vi "DataSetToVariantArrays.vi"() -> ()   [LabVIEW 2014, in "TableLogger_SQLite_Actor.lvlib" / "TableLogger_SQLite_Actor.lvclass"]
uses:
  TableLogger_SQLite_Actor.lvclass
  TableLogger_Actor/TableLogger_Actor/TableLogger_Actor.lvclass
panel:
  out "Data 2":variant[](array[variant])
  out "Data":string[](array[string])
  in  "LV Data":T1={"Numeric Data"=1245, "Float Data"=896.578, "String Data"="Tessolve", "Enum Data"=enum."Enum Item 2", "Array Data"=[8787, 457], "Cluster"={"String"="Hi", "Array Data 2"=[1, 2]}, "Array Data 2"=[3, 2, 1], "Cluster 2"={"String"="hello", "Array Data 2"=[1, 2]}, "Cluster 3"={"Cluster78"={"Array Data 2"=[987, 789]}}}
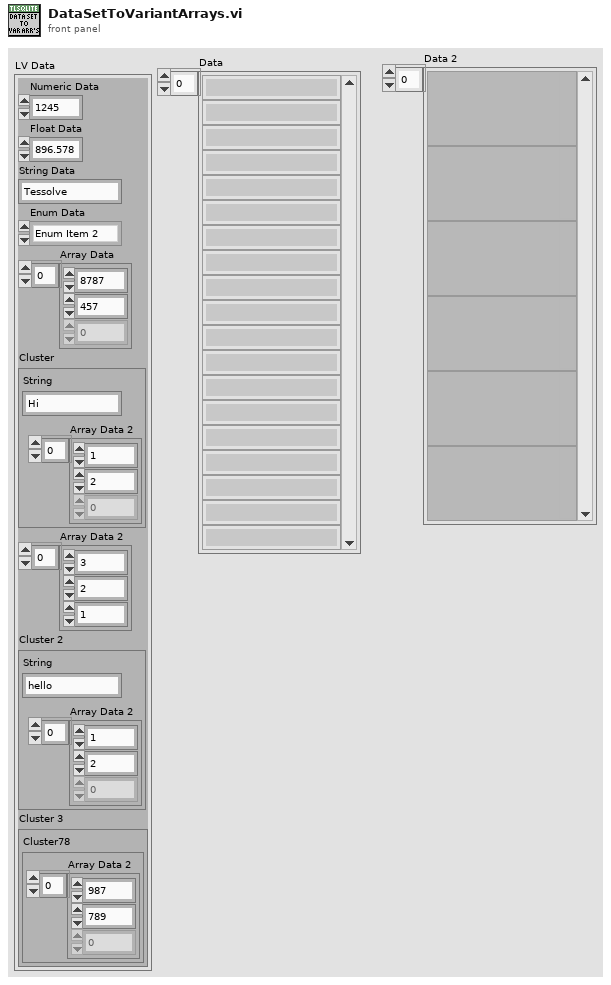
[diagram p1: front panel]
types:
  T1 = cluster{"Numeric Data":i32, "Float Data":dbl, "String Data":string, "Enum Data":enum16{"Enum Item 1", "Enum Item 2"}, "Array Data":i32[], "Cluster":cluster{"String":string, "Array Data 2":i32[]}, "Array Data 2":i32[], "Cluster 2":cluster{"String":string, "Array Data 2":i32[]}, "Cluster 3":cluster{"Cluster78":cluster{"Array Data 2":i32[]}}}
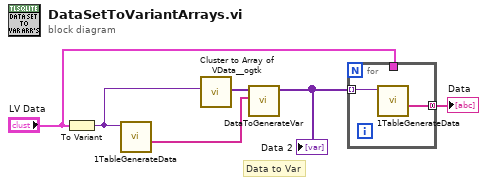
[diagram p0: block diagram]
diagram:
  # "Data to Var"
  n1 = To Variant(anything="LV Data") -> (Variant=w4:variant)
  n2 = call "1TableGenerateData.vi"("Cluster Variant"=w4) -> ("Data"=w2:string[])  [unwired: 6 in, 4 out]
  n3 = call <userlib>:"Cluster to Array of VData__ogtk.vi"("Cluster"=w4) -> ("Array of VData"=w3:variant[])  [unwired: 9 in, 1 out]
  n4 = call "DataToGenerateVar.vi"("Data in"=w2, "Array of VData"=w3) -> ("Data"=w5:variant[])  [unwired: 7 in, 2 out]
  "Data 2" <- w5
  n5 = for {
    tunnel: "LV Data" -> [_]
    tunnel: [w8] -> w1 mode=concatenating
    tunnel: w5 -> [w7] mode=indexing
    n6 = call "1TableGenerateData.vi"("Cluster Variant"=w7) -> ("Data"=w8:string[])  [unwired: 6 in, 4 out]
  }
  "Data" <- w1
